vi "AMI Responce Bytes Count.vi"() -> (0 "Bytes Count":u32)   [LabVIEW 2015, in "Samwontech TEMP2xxx.lvlib"]
uses:
  Samwontech TEMP2xxx.lvlib
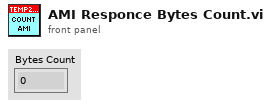
[diagram p1: front panel]
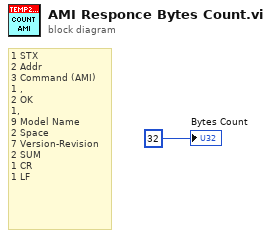
[diagram p0: block diagram]
diagram:
  # "1 STX\n2 Addr\n3 Command (AMI)\n1 ,\n2 OK\n1,\n9 Model Name\n2 Space\n7 Version-Revision\n2 SUM\n1 CR\n1 LF"
  "Bytes Count" <- u32 32
